vi "RTS Check Open TDMS.vi"(7 "Setup Info Station #":string[][](array[string]), 8 "error in (no error)":errorcluster, 9 "Data":string[][](array[string]), 10 "CSV File Location":path, 11 "Byte Stream File In":refnum<file>) -> (0 "error out":errorcluster, 2 "Open All CSV Data":bool, 3 "Byte Stream File Out":refnum<file>)   [LabVIEW 2020]
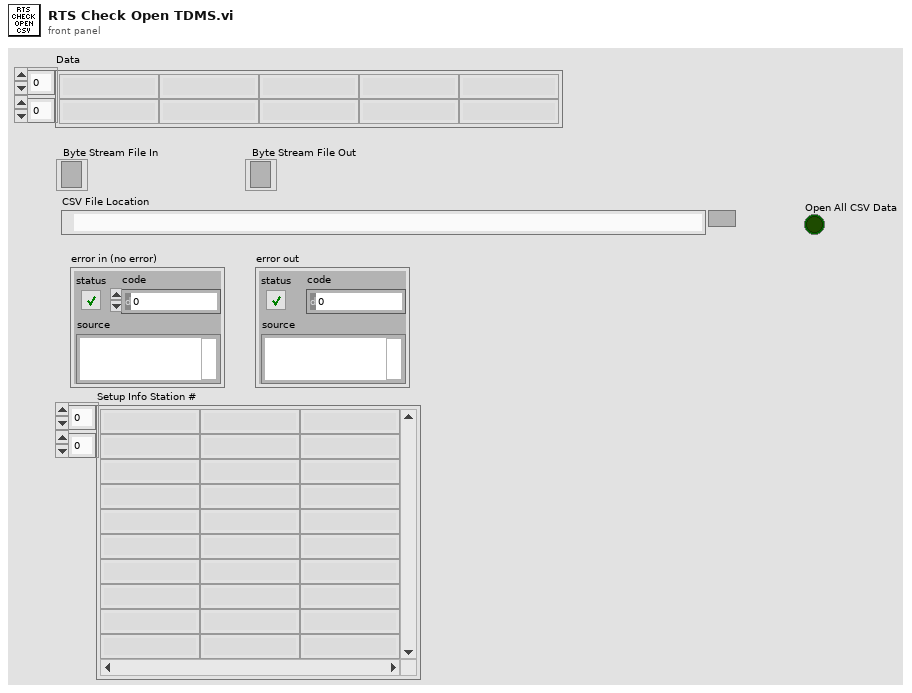
[diagram p1: front panel]
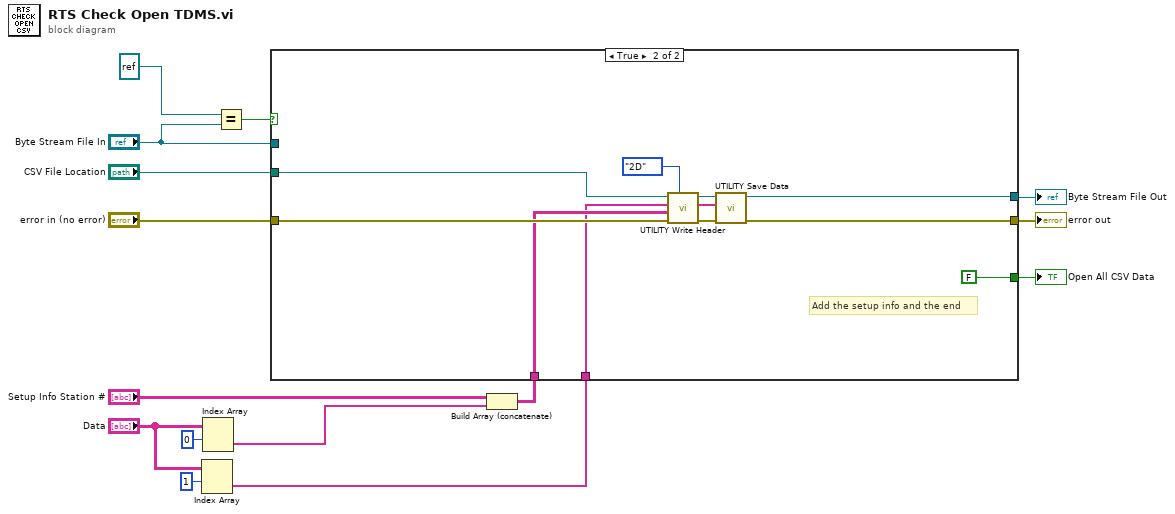
[diagram p0: block diagram]
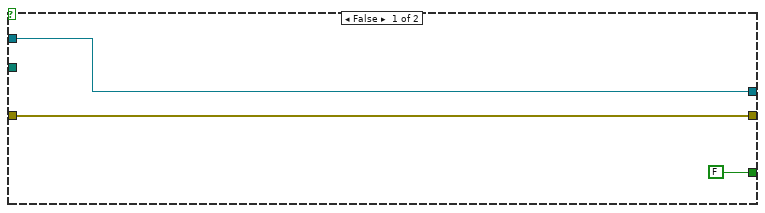
[diagram p2: hidden frame]
diagram:
  n1 = Index Array(array="Data", index (row)=1) -> (element=w5:string[])  [unwired: 1 in]
  n2 = Index Array(array="Data", index (row)=0) -> (element=w9:string[])  [unwired: 1 in]
  n3 = Equal?(x=refnum<file> refnum, y="Byte Stream File In") -> (x = y?=w4:bool)
  n4 = Build Array (concatenate)("Setup Info Station #", w9) -> (w8:string[][])
  n5 = case shown="True" w4 {
    tunnel: "error in (no error)" -> [w17 w28]
    tunnel: [w17 w27] -> w14
    tunnel: "CSV File Location" -> [_ w26]
    tunnel: [w18 w25] -> w1
    tunnel: "Byte Stream File In" -> [w18 _]
    tunnel: [FALSE FALSE] -> w12
    tunnel: w8 -> [_ w23]
    tunnel: w5 -> [_ w22]
    frame False {
    }
    frame True {
      # "Add the setup info and the end"
      n6 = call "UTILITY Write Header.vi"("Array Type"=enum16{"1D", "2D"}."2D", "error in (no error)"=w28, "Headers 2D"=w23, "File Path Control"=w26) -> ("error out"=w19:errorcluster, "Byte Stream File out"=w20:refnum<file>)  [unwired: 6 in]
      n7 = call "UTILITY Save Data.vi"("error in"=w19, "Data"=w22, "refnum"=w20) -> ("error out"=w27:errorcluster, "refnum out"=w25:refnum<file>)  [unwired: 7 in]
    }
  }
  "error out" <- w14
  "Open All CSV Data" <- w12
  "Byte Stream File Out" <- w1
